vi "Init.vi"(8 "error in (no error)":errorcluster, 11 "BetterListboxHandle in":refnum<class "BetterListboxHandle.lvclass">) -> (0 "error out":errorcluster, 3 "BetterListboxHandle out":refnum<class "BetterListboxHandle.lvclass">)   [LabVIEW 2020, in "BetterDragAndDrop.lvlib" / "BetterListboxHandle.lvclass"]
uses:
  BetterListboxHandle.lvclass
  C:/DSCE code/Open-source/betterdraganddrop_GIT/Source/Classes/BetterHandle/BetterHandle.lvclass
  BetterListboxHandle.lvclass/BetterListboxHandle.ctl
  BetterHandle/Pixel Constants.ctl
  BetterHandle/BetterHandle.lvclass/BetterHandle.ctl
  BetterHandle/Write Constant Sizes.vi
  BetterHandle/BetterHandle.lvclass
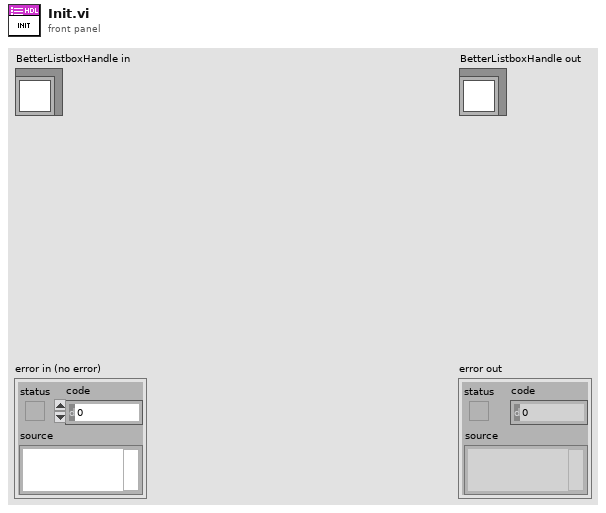
[diagram p1: front panel]
types:
  T1 = typedef "BetterDragAndDrop.lvlib/BetterHandle.lvclass/Pixel Constants.ctl" = cluster{"Row Header height":i32, "Row height":i32, "Column Header Offset":i32}
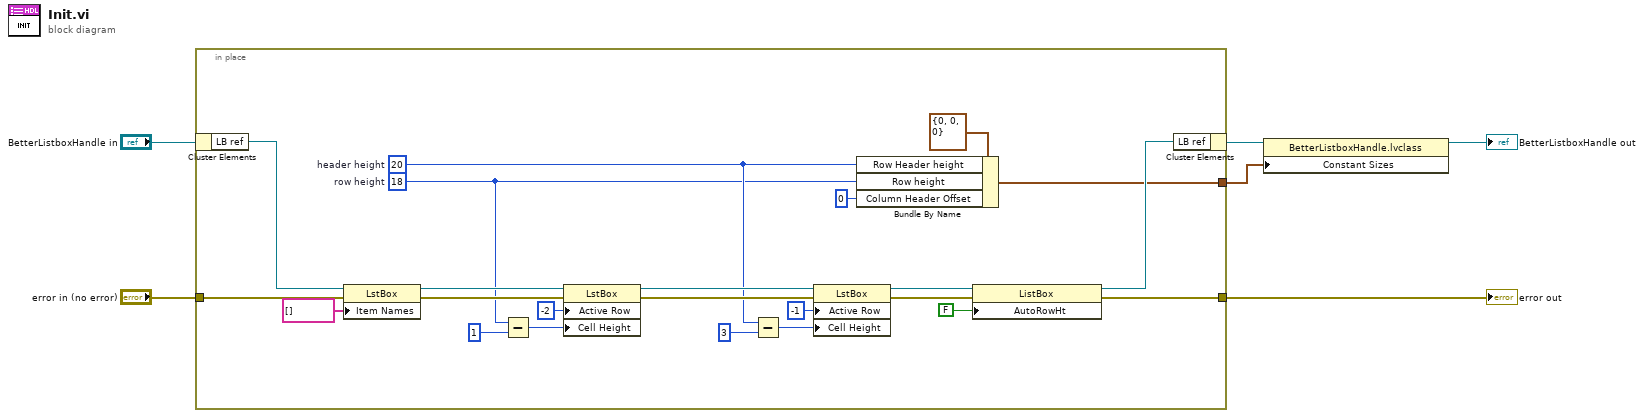
[diagram p0: block diagram]
diagram:
  n1 = in-place {
    in-place-border: "error in (no error)" -> [w28]
    in-place-border: [w13] -> w4
    in-place-border: [w7] -> w1
    w9 = 18  # row height
    w10 = 20  # header height
    n2 = in-place-cluster #1("BetterListboxHandle in") -> ("LB ref"=w29:refnum<vi>)
    n3 = property class="LstBox"(reference=w29, error in=w28, "Item Names"=string[] []) -> (reference out=w26:refnum<vi>, error out=w24:errorcluster)
    n4 = Subtract(x=w9, y=1) -> (x-y=w22:i32)
    n5 = property class="LstBox"(reference=w26, error in=w24, "Active Row"=-2 ("Active Row:Active Row Number"), "Cell Height"=w22) -> (reference out=w12:refnum<vi>, error out=w18:errorcluster)
    n6 = Subtract(x=w10, y=3) -> (x-y=w21:i32)
    n7 = property class="LstBox"(reference=w12, error in=w18, "Active Row"=-1 ("Active Row:Active Row Number"), "Cell Height"=w21) -> (reference out=w16:refnum<vi>, error out=w15:errorcluster)
    n8 = Bundle By Name(cluster=T1 {"Row Header height"=0, "Row height"=0, "Column Header Offset"=0} ("Constant Sizes"), "Row Header height"=w10, "Row height"=w9, "Column Header Offset"=0) -> (w7:T1)
    n9 = property class="ListBox"(reference=w16, error in=w15, "AutoRowHt"=FALSE ("Autosizing Row Height")) -> (reference out=w14:refnum<vi>, error out=w13:errorcluster)
    n10 = in-place-cluster #1("LB ref"=w14) -> (w3:refnum<class "BetterListboxHandle.lvclass">)
  }
  "error out" <- w4
  n11 = property class="BetterListboxHandle.lvclass"(reference=w3, "Constant Sizes"=w1) -> (reference out=→"BetterListboxHandle out":refnum<class "BetterListboxHandle.lvclass">)  [unwired: 1 in, 1 out]
